vi "ControlValueLoad.vi"(6 "ファイル名入力?(f)":bool, 8 "err(in)":errorcluster, 11 "VI refnum":refnum<vi>) -> (0 "err(out)":errorcluster)   [LabVIEW 2014]
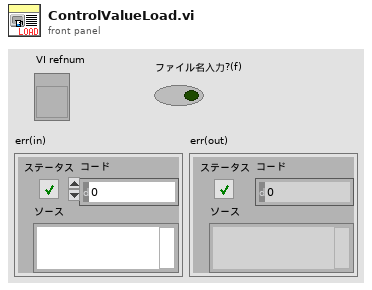
[diagram p1: front panel]
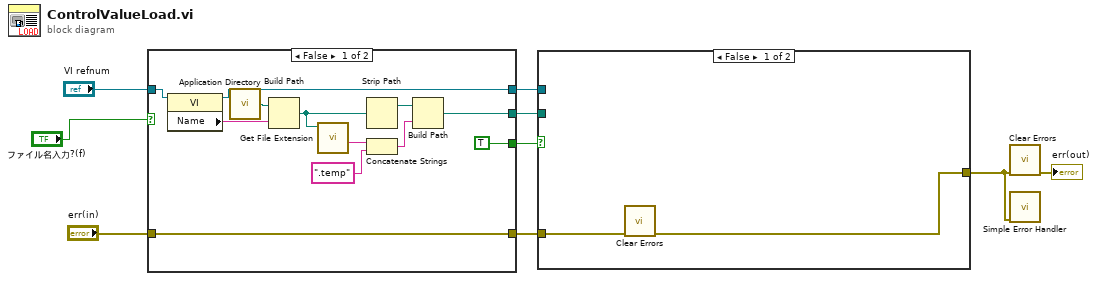
[diagram p0: block diagram]
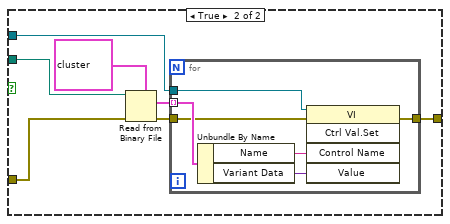
[diagram p2: hidden frame]
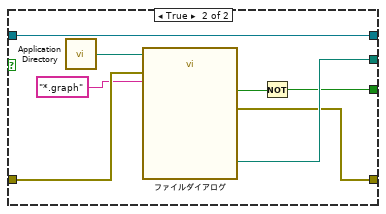
[diagram p3: hidden frame]
diagram:
  n1 = case shown="FALSE" "ファイル名入力?(f)" {
    tunnel: [w21 w29] -> w7
    tunnel: "VI refnum" -> [w20 w28]
    tunnel: [w19 w28] -> w5
    tunnel: [w11 w24] -> w2
    tunnel: "err(in)" -> [w11 w27]
    tunnel: [TRUE w25] -> w1
    frame False {
      n2 = property class="VI"(reference=w20) -> (reference out=w19:refnum<vi>, "Name"=w17:string)  [unwired: 1 in, 1 out]
      n3 = call <vilib>:"Application Directory.vi"() -> ("Application Directory"=w18:path)
      n4 = Build Path(base path=w18, name or relative path=w17) -> (appended path=w12:path)
      n5 = call <vilib>:"Get File Extension.vi"("file"=w12) -> ("filename without extension"=w15:string)  [unwired: 7 in, 3 out]
      n6 = Strip Path(path=w12) -> (stripped path=w16:path)  [unwired: 1 out]
      n7 = Concatenate Strings(w15, ".temp" ("名前または相対パス")) -> (w13:string)
      n8 = Build Path(base path=w16, name or relative path=w13) -> (appended path=w21:path)
    }
    frame True {
      n9 = call <vilib>:"Application Directory.vi"() -> ("Application Directory"=w23:path)
      n10 = call "ファイルダイアログ"("start path"=w23, "error in"=w27, "pattern (all files)"="*.graph") -> ("selected path"=w29:path, "cancelled"=w26:bool, "error out"=w24:errorcluster)  [unwired: 9 in, 1 out]
      n11 = Not(x=w26) -> (.not. x?=w25:bool)
    }
  }
  n12 = case shown="FALSE" w1 {
    tunnel: [w30 w38] -> w8
    tunnel: w7 -> [_ w37]
    tunnel: w5 -> [_ w36]
    tunnel: w2 -> [w31 w32]
    frame False {
      n13 = call <vilib>:"Clear Errors.vi"("error in (no error)"=w31) -> ("error out"=w30:errorcluster)  [unwired: 5 in, 1 out]
    }
    frame True {
      n14 = Read from Binary File(5:cluster{"Name":string, "Variant Data":variant}[] [{"Name"="数値", "Variant Data"=variant(dbl 2.0)}, {"Name"="ブール", "Variant Data"=variant(bool FALSE)}, {"Name"="文字列", "Variant Data"=variant(string "")}] ("制御器の値 2"), 8:w32, 11:w37) -> (0:w33:errorcluster, 2:w35:cluster{"Name":string, "Variant Data":variant}[])  [unwired: 3 in, 2 out]
      n15 = for {
        tunnel: w35 -> [w44] mode=indexing
        tunnel: w36 -> [w43]
        tunnel: w33 -> [w40]
        tunnel: [w39] -> w38
        n16 = Unbundle By Name(w44) -> ("Name"=w42:string, "Variant Data"=w41:variant)
        n17 = invoke class="VI" method="Ctrl Val.Set"(reference=w43, error in=w40, "Control Name"=w42, "Value"=w41) -> (error out=w39:errorcluster)  [unwired: 1 in, 4 out]
      }
    }
  }
  n18 = call <vilib>:"Clear Errors.vi"("error in (no error)"=w8) -> ("error out"=→"err(out)":errorcluster)  [unwired: 5 in, 1 out]
  n19 = call <vilib>:"Simple Error Handler.vi"("error in (no error)"=w8) -> ()  [unwired: 4 in, 5 out]
